vi "ad2xy.vi"(8 "DEC":dbl format="%.6g", 9 "RA":dbl format="%.6g", 11 "Astrometry":T1 {"CRVAL" format="%.6g"; "CD" format="%_8g"; "NAXIS" format="%.6g"}) -> (0 "Y":dbl, 1 "X":dbl, 3 "Dup Astrometry":T1 {"CRVAL" format="%.6g"; "CD" format="%_7g"})   [LabVIEW 2019]
uses:
  <vilib>/Analysis/Matrix/Numeric/Conversions/Array To Matrix - RA2.vi
  <vilib>/Analysis/baseanly.llb/Real Inverse Matrix.vi
  <vilib>/Analysis/Matrix/Numeric/Conversions/Matrix To Array - RM.vi
  <vilib>/Analysis/Matrix/NI_Matrix.lvlib
  <vilib>/Analysis/NI_AALBase.lvlib
panel:
  out "DEC (CRVAL)":dbl format="%<%H:%M:%S%1u>t"
  out "RA (CRVAL)":dbl format="%<%H:%M:%S%2u>t"
  out "ydif":dbl
  out "xdif":dbl
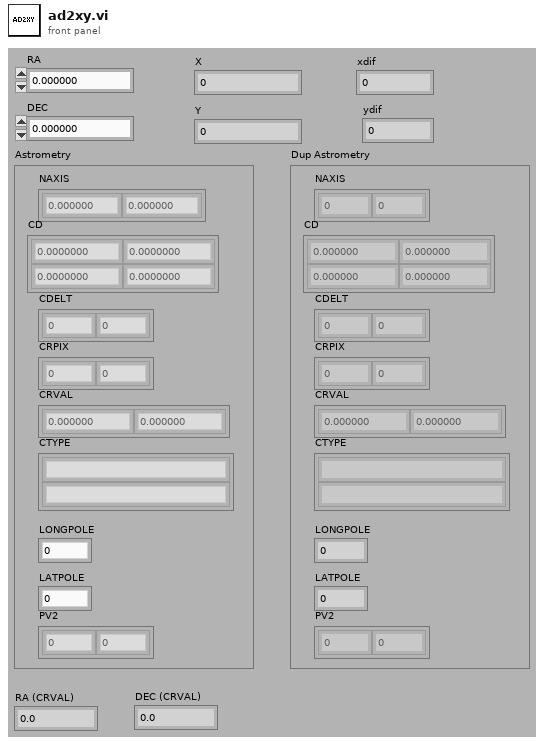
[diagram p1: front panel]
types:
  T1 = cluster{"NAXIS":dbl[], "CD":dbl[][], "CDELT":dbl[], "CRPIX":dbl[], "CTYPE":string[], "CRVAL":dbl[], "LONGPOLE":dbl, "LATPOLE":dbl, "PV2":dbl[]}
  T2 = typedef "NI_Matrix.lvlib/RealMatrix.ctl" = dbl[][]
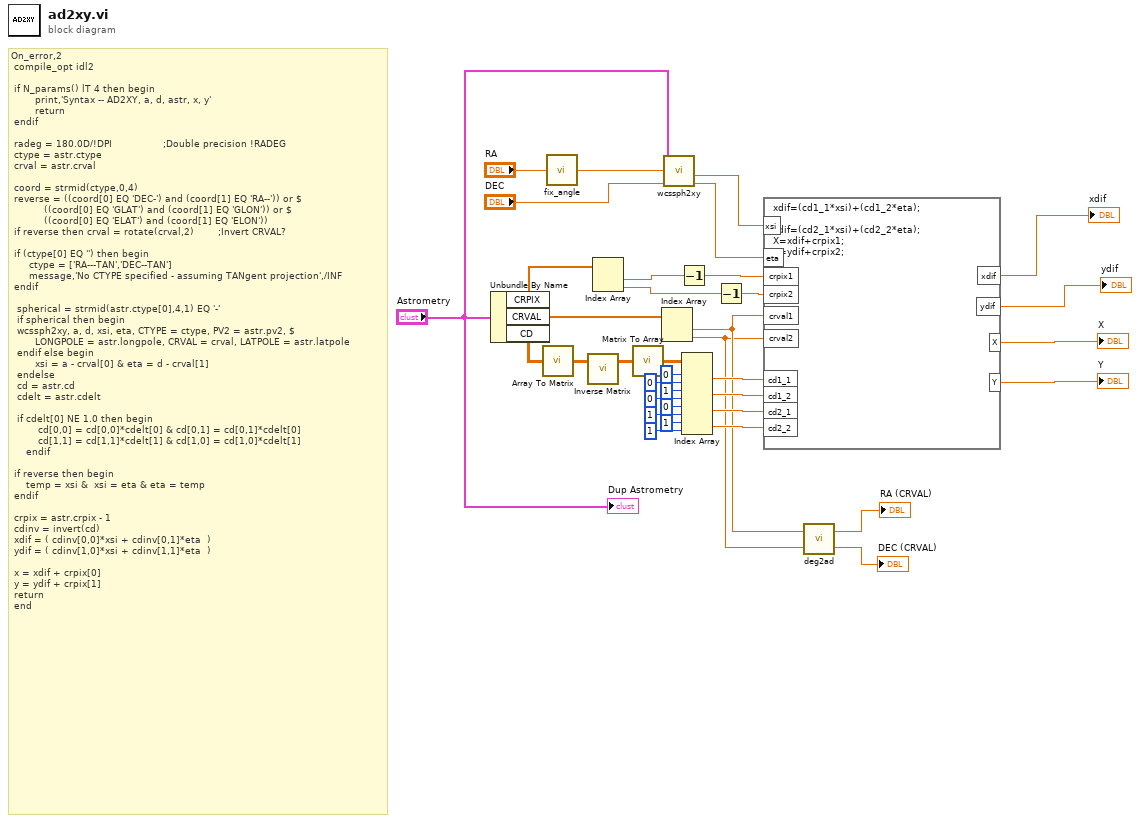
[diagram p0: block diagram]
diagram:
  # "On_error,2\n compile_opt idl2\n\n if N_params() lT 4 then begin\n        print,'Syntax -- AD2XY, a, d, astr, x, y'\n        return\n endif\n\n radeg = 180.0D/!DPI                 ;Double precision !RADEG\n ctype = astr.ctype\n crval = astr.crval\n\n coord = strmid(ctype,0,4)\n reverse = ((coord[0] EQ 'DEC-') and (coord[1] EQ 'RA--')) or $\n           ((coord[0] EQ 'GLAT') and (coord[1] EQ 'GLON')) or $\n           ((coord[0] EQ 'ELAT') and (coord[1] EQ 'ELON'))\n if reverse then crval = rotate(crval,2)        ;Invert CRVAL?\n\n if (ctype[0] EQ '') then begin   \n      ctype = ['RA---TAN','DEC--TAN']\n      message,'No CTYPE specified - assuming TANgent projection',/INF\n endif      \n     \n  spherical = strmid(astr.ctype[0],4,1) EQ '-'\n  if spherical then begin\n  wcssph2xy, a, d, xsi, eta, CTYPE = ctype, PV2 = astr.pv2, $\n        LONGPOLE = astr.longpole, CRVAL = crval, LATPOLE = astr.latpole\n  endif else begin\n        xsi = a - crval[0] & eta = d - crval[1]\n  endelse\t\n  cd = astr.cd\n  cdelt = astr.cdelt\n\n  if cdelt[0] NE 1.0 then begin\n         cd[0,0] = cd[0,0]*cdelt[0] & cd[0,1] = cd[0,1]*cdelt[0]\n         cd[1,1] = cd[1,1]*cdelt[1] & cd[1,0] = cd[1,0]*cdelt[1]\n     endif\n\n if reverse then begin\n     temp = xsi &  xsi = eta & eta = temp\n endif\n\n crpix = astr.crpix - 1\n cdinv = invert(cd)\n xdif = ( cdinv[0,0]*xsi + cdinv[0,1]*eta  )\n ydif = ( cdinv[1,0]*xsi + cdinv[1,1]*eta  )\n\n x = xdif + crpix[0] \n y = ydif + crpix[1] \n return\n end"
  n1 = Unbundle By Name("Astrometry") -> ("CRPIX"=w31:dbl[], "CRVAL"=w34:dbl[], "CD"=w36:dbl[][])
  n2 = call-poly <vilib>:"Array To Matrix.vi"("Real 2D Array"=w36) -> ("Real Matrix"=w35:T2)
  n3 = call "fix_angle.vi"("Angle IN"="RA") -> ("Angle OUT"=w14:dbl)  [unwired: 4 in]
  n4 = call-poly <vilib>:"Inverse Matrix.vi"("Input Matrix"=w35) -> ("Inverse Matrix"=w30:T2)  [unwired: 1 in, 1 out]
  n5 = Index Array(array=w31) -> (element #1=w33:dbl, element #2=w32:dbl)  [unwired: 2 in]
  n6 = call-poly <vilib>:"Matrix To Array.vi"("Real Matrix"=w30) -> ("Real 2D Array"=w29:dbl[][])
  n7 = Index Array(array=w34) -> (element #1=w4:dbl, element #2=w3:dbl)  [unwired: 2 in]
  n8 = call "wcssph2xy.vi"("lat"="DEC", "lon"=w14, "Astrometry"="Astrometry") -> ("Y"=w11:dbl, "X"=w12:dbl)  [unwired: 7 in]
  n9 = Decrement(x=w33) -> (x-1=w10:dbl)
  n10 = Index Array(array=w29, index (row) #1=0 ("index (row)"), index (col) #1=0 ("disabled index (col)"), index (row) #2=1 ("index (row)"), index (col) #2=0 ("disabled index (col)"), index (row) #3=0 ("index (row)"), index (col) #3=1 ("disabled index (col)"), index (row) #4=1 ("index (row)"), index (col) #4=1 ("disabled index (col)")) -> (element #1=w20:dbl, element #2=w19:dbl, element #3=w18:dbl, element #4=w17:dbl)
  n11 = Decrement(x=w32) -> (x-1=w9:dbl)
  n12 = formula code="xdif=(cd1_1*xsi)+(cd1_2*eta);\n\nydif=(cd2_1*xsi)+(cd2_2*eta);\nX=xdif+crpix1;\nY=ydif+crpix2;"("xsi"=w12, "eta"=w11, "crval1"=w4, "crval2"=w3, "cd1_1"=w20, "crpix1"=w10, "crpix2"=w9, "cd1_2"=w19, "cd2_1"=w18, "cd2_2"=w17) -> ("xdif"=→"xdif":dbl, "ydif"=→"ydif":dbl, "X"=→"X":dbl, "Y"=→"Y":dbl)
  n13 = call "deg2ad.vi"("DEC (°)"=w3, "RA (°)"=w4) -> ("DEC (°)"=→"DEC (CRVAL)":dbl, "RA (sec)"=→"RA (CRVAL)":dbl)
  "Dup Astrometry" <- "Astrometry"
